vi "run_auto_test M.vi"(7 "Cluster":T1, 8 "error in (no error)":errorcluster) -> (0 "error out":errorcluster)   [LabVIEW 2019]
uses:
  core_dataRefCluster.ctl
  core_dataRef.ctl
  core_dataCluster.ctl
  instrument/instr_dataCluster.ctl
  instrument/Instrument.lvclass
panel:
  in  "modbusData":refnum<notifier>
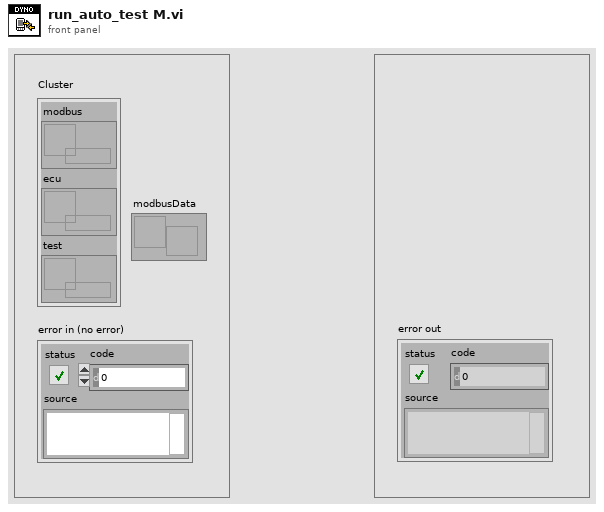
[diagram p1: front panel]
types:
  T1 = typedef "core_dataRefCluster.ctl" = cluster{"modbus":T2, "ecu":T2, "test":T2}
  T2 = typedef "core_dataRef.ctl" = refnum<queue>
  T3 = typedef "core_dataCluster.ctl" = cluster{"cmd":string, "data":variant}
  T4 = typedef "Instrument.lvclass/instr_dataCluster.ctl" = cluster{"电源电压 V":dbl, "电源电流A":dbl, "扭矩N/m":dbl, "速度r/M":dbl, "温度℃":dbl[], "流量计L/M":dbl[]}
  T5 = typedef "ecu_dataCluster.ctl" = cluster{"MCU_MotCtrlrSts":dbl, "MCU_MotTq":dbl, "MCU_MotBusU":dbl, "MCU_MotSpd":dbl, "MCU_MotBodyT":dbl, "MCU_MotBody_T":dbl, "MCU_MotCtrlrT":dbl, "MCU 状态":bool, "ErrMsg":i64}
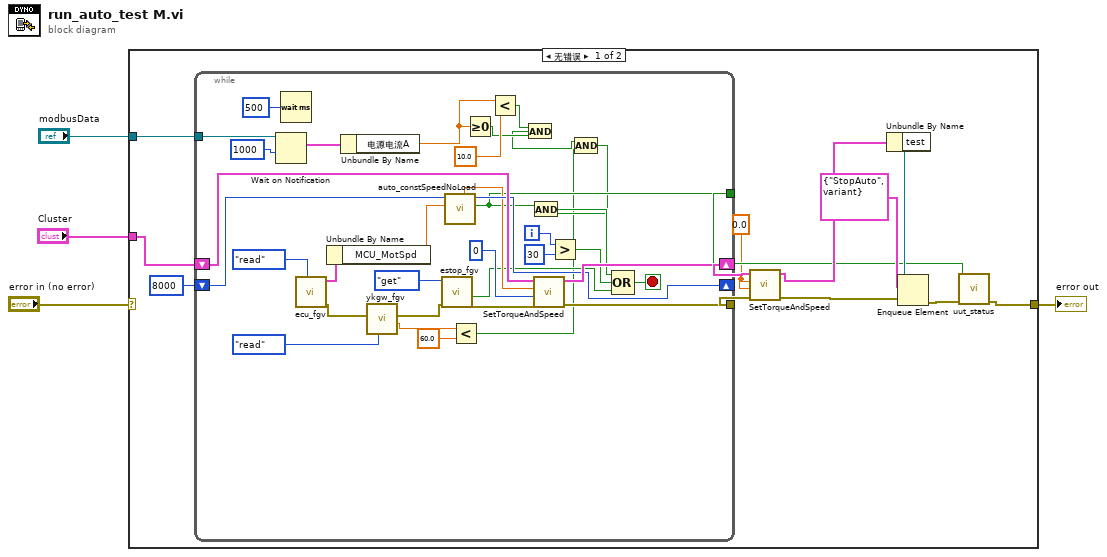
[diagram p0: block diagram]
diagram:
  n1 = case shown="无错误" "error in (no error)" {
    selector: "error in (no error)" -> [_ w53]
    tunnel: "Cluster" -> [w17 _]
    tunnel: [w5 w53] -> w3
    tunnel: "modbusData" -> [w11 _]
    frame No Error {
      w7 = sgl 0.0 ("Torque")
      n2 = while {
        shift-right: [w51] -> w15
        shift-left: w17 -> [w52]
        shift-right: [w48] -> _
        shift-left: 8000 ("Speed") -> [w50]
        tunnel: [w30] -> w8
        tunnel: [w42] -> w12
        tunnel: w11 -> [w35]
        i -> [w47]
        stop <- w31 stop-if-true
        n3 = Wait on Notification(notifier=w35, timeout in ms (-1)=1000 ("超时毫秒(-1)")) -> (notification=w33:T4)  [unwired: 2 in, 3 out]
        n4 = Wait (ms)(milliseconds to wait=u32 500) -> ()  [unwired: 1 out]
        n5 = call "ecu_fgv.vi"("mode"=enum16{"read", "write"}."read") -> ("error out"=w28:errorcluster, "data out"=w41:T5)  [unwired: 9 in]
        n6 = Unbundle By Name(w41) -> ("MCU_MotSpd"=w49:dbl)
        n7 = Unbundle By Name(w33) -> ("电源电流A"=w18:dbl)
        n8 = call "ykgw_fgv.vi"("mode"=enum16{"read", "write"}."read", "error in (no error)"=w28) -> ("phase current"=w19:dbl, "error out"=w27:errorcluster)  [unwired: 5 in, 3 out]
        n9 = call "estop_fgv.vi"("error in (no error)"=w27, "Enum"=enum16{"set", "get"}."get") -> ("error out"=w36:errorcluster, "indicator"=w37:bool)  [unwired: 8 in]
        n10 = call "auto_constSpeedNoLoad.vi"("speed"=w49, "Speed"=w50) -> ("Pass"=w30:bool, "Set speed"=w48:i32, "torque"=w44:sgl)  [unwired: 7 in]
        n11 = Less?(x=w19, y=60.0) -> (x < y?=w21:bool)
        n12 = Greater Or Equal To 0?(x=w18) -> (x >= 0?=w22:bool)
        n13 = Less?(x=w18, y=10.0) -> (x < y?=w23:bool)
        n14 = And(x=w23, y=w22) -> (x .and. y?=w20:bool)
        n15 = call "SetTorqueAndSpeed.vi"("error in (no error)"=w36, "Speed"=0, "Torque"=w44, "Cluster in"=w52) -> ("error out"=w42:errorcluster, "Cluster out"=w51:T1)  [unwired: 6 in]
        n16 = Greater?(x=w47, y=30) -> (0:w45:bool)
        n17 = Compound Arithmetic op=AND(w20, w21) -> (w25:bool)
        n18 = And(x=w30, y=w25) -> (x .and. y?=w32:bool)
        n19 = Compound Arithmetic op=OR(w32, w45, w37) -> (w31:bool)
      }
      n20 = call "SetTorqueAndSpeed.vi"("error in (no error)"=w12, "Speed"=w7, "Torque"=w7, "Cluster in"=w15) -> ("error out"=w6:errorcluster, "Cluster out"=w10:T1)  [unwired: 6 in]
      n21 = Unbundle By Name(w10) -> ("test"=w14:T2)
      n22 = Enqueue Element(queue=w14, element=T3 {"cmd"="StopAuto", "data"=variant}, error in (no error)=w6) -> (error out=w9:errorcluster)  [unwired: 1 in, 2 out]
      n23 = call "uut_status.vi"("error in (no error)"=w9, "status"=w8) -> ("error out"=w5:errorcluster)  [unwired: 9 in]
    }
    frame Error {
    }
  }
  "error out" <- w3
